vi "Version_Check.vi"(0 "GEA2 Reference In":refnum<k24>, 1 "Verify?":bool, 2 "Standalone?":bool, 5 "GEA Inputs":T1={"Source"=228, "Destination"=35} {"Destination" format="%.0x"; "Source" format="%.0x"}, 7 "Expected Application Version":string, 9 "Expected Parametric Version":string, 11 "Error In":errorcluster) -> (4 "GEA2 Reference Out":refnum<k24>, 6 "Pass/Fail?":bool, 8 "Actual Application Version":string, 10 "Actual Parametric Version":string, 14 "Report Text":string, 15 "Error Out":errorcluster)   [LabVIEW 2016]
doc: "This VI takes the user's input of expected application and parametric software versions and compares them to the actual software present via ERD query"
uses:
  Q:/Common/DLLs/GEA3/GeaCommunication.dll
  Common/DLLs/GEA3/GeaCommunication.dll
  Common/LabVIEW GEA2 Toolkit/LabVIEW_GEA2_Toolkit.lvlibp/type defs/Source_Destination.ctl
  Common/LabVIEW GEA2 Toolkit/LabVIEW_GEA2_Toolkit.lvlibp/type defs/ERD Read Data In.ctl
  Common/LabVIEW GEA2 Toolkit/LabVIEW_GEA2_Toolkit.lvlibp/type defs/Data Type.ctl
  Common/LabVIEW GEA2 Toolkit/LabVIEW_GEA2_Toolkit.lvlibp
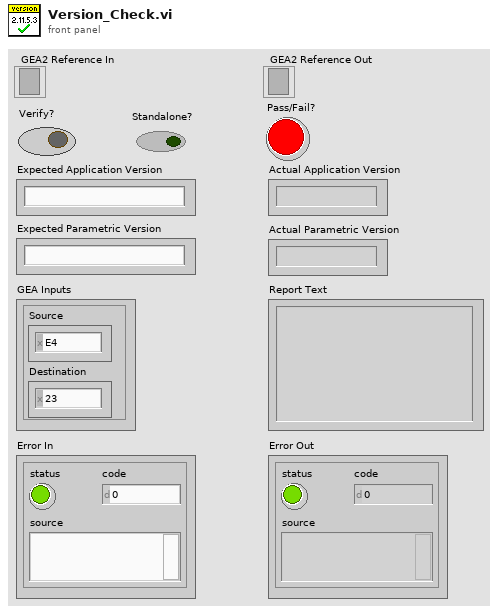
[diagram p1: front panel]
types:
  T1 = typedef "LabVIEW_GEA2_Toolkit.lvlibp/Source_Destination.ctl" = cluster{"Source":u8, "Destination":u8}
  T2 = typedef "LabVIEW_GEA2_Toolkit.lvlibp/ERD Read Data In.ctl" = cluster{"ERD Number":u16, "Data Type":T3}
  T3 = typedef "LabVIEW_GEA2_Toolkit.lvlibp/Data Type.ctl" = enum16{"string", "boolean", "uint8_t", "uint16_t", "uint32_t", "uint64_t", "int8_t", "int16_t", "int32_t", "int64_t"}
  T4 = typedef "LabVIEW_GEA2_Toolkit.lvlibp/ERD Read Data Out.ctl" = cluster{"ERD Number":u16, "Data":string}
  T5 = cluster{"[0]":string, "[1]":string, "[2]":string, "[3]":string, "[4]":string, "[5]":string, "[6]":string, "[7]":string, "[8]":string}
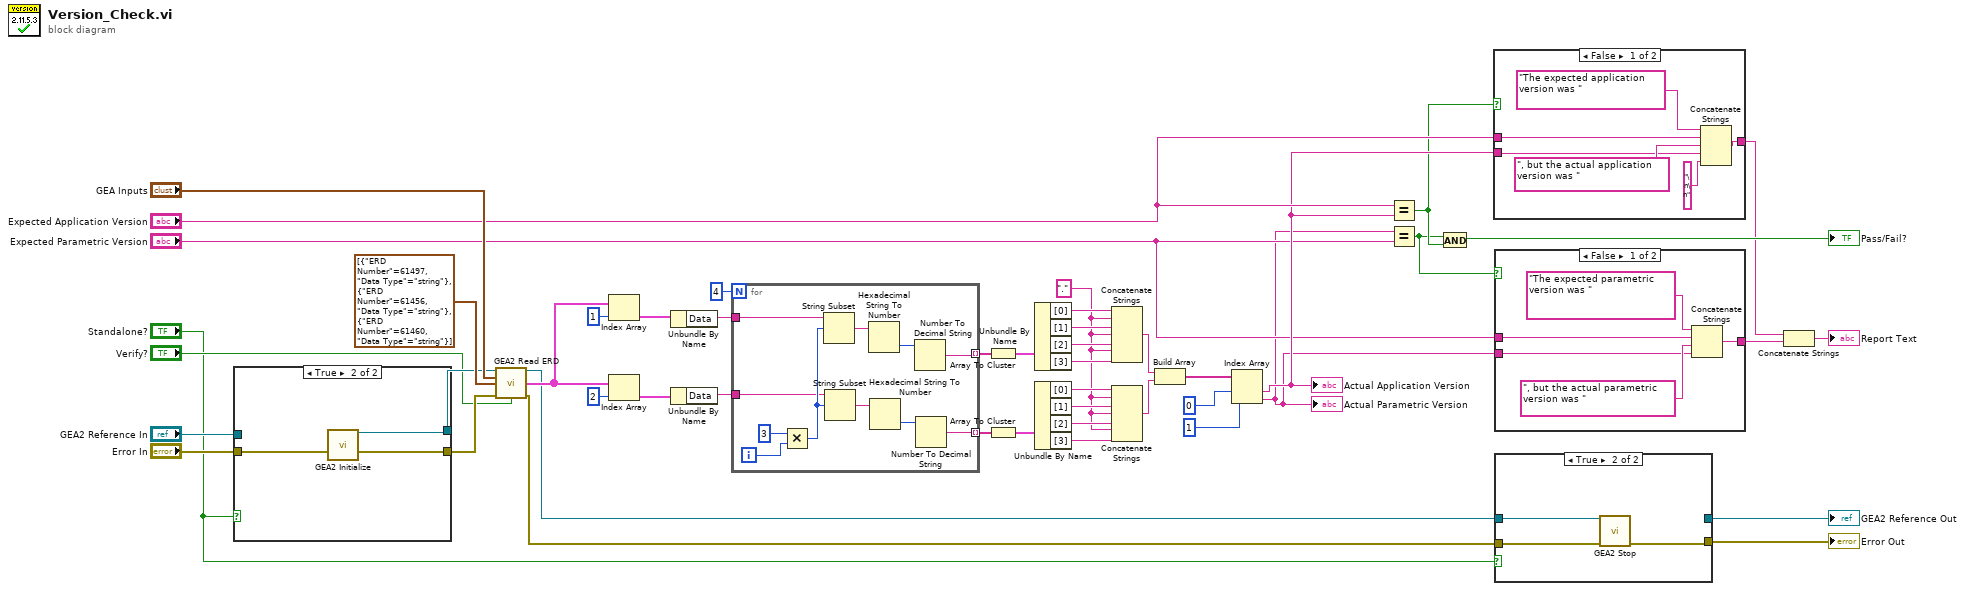
[diagram p0: block diagram]
diagram:
  w20 = "." ("string")
  n1 = case shown="True" "Standalone?" {
    tunnel: [w50 w52] -> w45
    tunnel: "Error In" -> [w50 w53]
    tunnel: [w49 w51] -> w42
    tunnel: "GEA2 Reference In" -> [w49 _]
    frame False {
    }
    frame True {
      n2 = call "GEA2 Initialize.vi"("error in"=w53) -> ("GEA2 Reference Out"=w51:refnum<k24>, "error out"=w52:errorcluster)  [unwired: 12 in, 1 out]
    }
  }
  n3 = call "GEA2 Read ERD.vi"("GEA2 Reference In"=w42, "GEA Inputs"="GEA Inputs", "Read ERD List"=T2[] [{"ERD Number"=61497, "Data Type"=enum."string"}, {"ERD Number"=61456, "Data Type"=enum."string"}, {"ERD Number"=61460, "Data Type"=enum."string"}], "Error In"=w45, "Verify ERD Response?"="Verify?") -> ("GEA2 Reference Out"=w14:refnum<k24>, "ERD Data Out"=w39:T4[], "Error Out"=w15:errorcluster)  [unwired: 7 in, 1 out]
  n4 = Index Array(array=w39, index=1) -> (element=w38:T4)
  n5 = Index Array(array=w39, index=2) -> (element=w35:T4)
  n6 = Unbundle By Name(w38) -> ("Data"=w33:string)
  n7 = Unbundle By Name(w35) -> ("Data"=w19:string)
  n8 = for {
    N: 4 -> [_]
    tunnel: w33 -> [w61]
    tunnel: [w59] -> w32 mode=indexing
    tunnel: [w55] -> w21 mode=indexing
    tunnel: w19 -> [w54]
    i -> [w64]
    n9 = Multiply(x=3, y=w64) -> (x*y=w56:i32)
    n10 = String Subset(string=w61, offset (0)=w56) -> (substring=w62:string)  [unwired: 1 in]
    n11 = String Subset(string=w54, offset (0)=w56) -> (substring=w57:string)  [unwired: 1 in]
    n12 = Hexadecimal String To Number(string=w62) -> (number=w60:u32)  [unwired: 2 in, 1 out]
    n13 = Hexadecimal String To Number(string=w57) -> (number=w58:u32)  [unwired: 2 in, 1 out]
    n14 = Number To Decimal String(number=w60) -> (decimal integer string=w59:string)  [unwired: 1 in]
    n15 = Number To Decimal String(number=w58) -> (decimal integer string=w55:string)  [unwired: 1 in]
  }
  n16 = Array To Cluster(array=w32) -> (cluster=w31:T5)
  n17 = Array To Cluster(array=w21) -> (cluster=w22:T5)
  n18 = Unbundle By Name(w31) -> ("[0]"=w30:string, "[1]"=w29:string, "[2]"=w28:string, "[3]"=w27:string)
  n19 = Unbundle By Name(w22) -> ("[0]"=w23:string, "[1]"=w24:string, "[2]"=w25:string, "[3]"=w26:string)
  n20 = Concatenate Strings(w30, w20, w29, w20, w28, w20, w27) -> (w18:string)
  n21 = Concatenate Strings(w23, w20, w24, w20, w25, w20, w26) -> (w17:string)
  n22 = Build Array(w18, w17) -> (w13:string[])
  n23 = Index Array(array=w13, index #1=0 ("index"), index #2=1 ("index")) -> (element #1=w8:string, element #2=w4:string)
  "Actual Application Version" <- w8
  "Actual Parametric Version" <- w4
  n24 = Equal?(x="Expected Application Version", y=w8) -> (x = y?=w7:bool)
  n25 = Equal?(x=w4, y="Expected Parametric Version") -> (x = y?=w6:bool)
  n26 = And(x=w6, y=w7) -> (x .and. y?=→"Pass/Fail?":bool)
  n27 = case shown="False" w7 {
    tunnel: "Expected Application Version" -> [w68 _]
    tunnel: w8 -> [w67 _]
    tunnel: [w66 _] -> w2
    frame False {
      n28 = Concatenate Strings("The expected application version was " ("string"), w68, ", but the actual application version was " ("string"), w67, "\n\n" ("string")) -> (w66:string)
    }
    frame True {
    }
  }
  n29 = case shown="False" w6 {
    tunnel: "Expected Parametric Version" -> [w74 _]
    tunnel: w4 -> [w72 _]
    tunnel: [w71 _] -> w3
    frame False {
      n30 = Concatenate Strings("The expected parametric version was " ("string"), w74, ", but the actual parametric version was " ("string"), w72) -> (w71:string)
    }
    frame True {
    }
  }
  n31 = case shown="True" "Standalone?" {
    tunnel: [w77 w79] -> w48
    tunnel: w15 -> [w77 w80]
    tunnel: w14 -> [w76 w78]
    tunnel: [w76 _] -> w41
    frame False {
    }
    frame True {
      n32 = call "GEA2 Stop.vi"("GEA2 Reference In"=w78, "Error In"=w80) -> ("Error Out"=w79:errorcluster)  [unwired: 13 in]
    }
  }
  "GEA2 Reference Out" <- w41
  "Error Out" <- w48
  n33 = Concatenate Strings(w2, w3) -> (→"Report Text":string)
